vi "Process File.vi"(8 "error in (no error)":errorcluster, 10 "File":path, 11 "Format Converter in":refnum<class "Format Converter.lvclass">) -> (0 "error out":errorcluster, 2 "File out":path, 3 "Format Converter out":refnum<class "Format Converter.lvclass">)   [LabVIEW 2016, in "Format Converter.lvclass"]
uses:
  Format Converter.lvclass
  Read Format Converter Configuration.vi
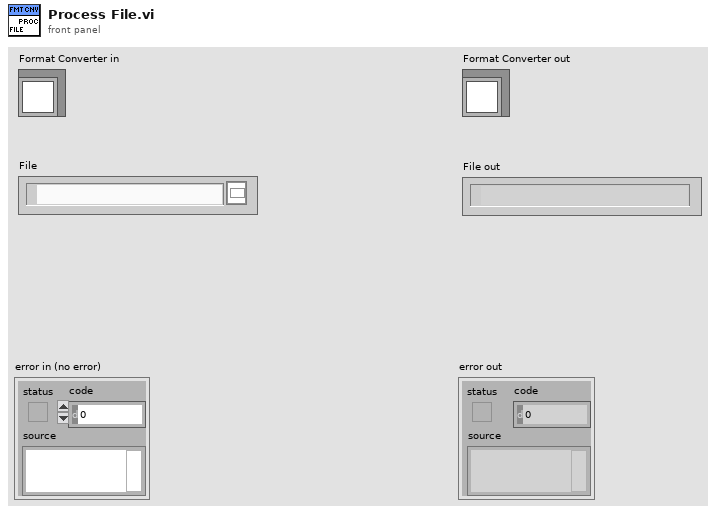
[diagram p1: front panel]
types:
  T1 = typedef "Format Converter Configuration.ctl" = cluster{"New start time":dbl, "New end time":dbl, "Output file format":enum16{"ASCII", "BINARY", "TDMS"}, "Save ASCII column names":bool, "Prepend binary array size":bool, "buffer size (-1: all)":i64, "Channels":string[], "Group":string, "New dt":dbl}
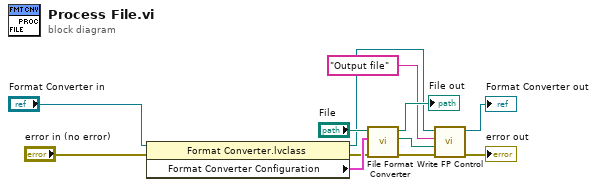
[diagram p0: block diagram]
diagram:
  n1 = property class="Format Converter.lvclass"(reference="Format Converter in", error in="error in (no error)") -> (reference out=w6:refnum<class "Format Converter.lvclass">, error out=w8:errorcluster, "Format Converter Configuration"=w9:T1)
  n2 = call "File Format Converter.vi"("Error In"=w8, "Configuration"=w9, "File"="File") -> ("Error Out"=w4:errorcluster, "New file out"=w2:path, "File out"=→"File out":path)  [unwired: 6 in]
  n3 = call-dynamic "Write FP Control.vi"("error in (no error)"=w4, "Control Value"=w2, "Control Name"="Output file", "Measure Object in"=w6) -> ("error out"=→"error out":errorcluster, "Measure Object out"=→"Format Converter out":refnum<class "Format Converter.lvclass">)  [unwired: 6 in]
